vi "test_mergeClusters.vi"(8 "error in (no error)":errorcluster) -> (0 "error out":errorcluster)   [LabVIEW 2020]
uses:
  _built_ppls/OpenVariant.lvlibp
  <vilib>/addons/_JKI Toolkits/Caraya/classes/Test/Test.lvclass
  <vilib>/addons/_JKI Toolkits/Caraya/classes/Assert/Assert.lvclass
  <vilib>/addons/_JKI Toolkits/Caraya/classes/Assert/Assert Equal Value and Type_Variant.vi
panel:
  out "Data out":variant
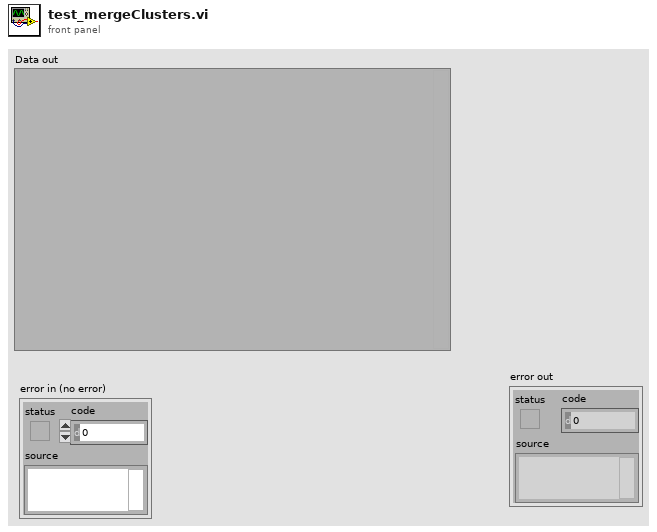
[diagram p1: front panel]
types:
  T1 = cluster{"status":bool, "source":string, "error":errorcluster}
  T2 = cluster{"status":bool, "source":string, "error":cluster{"status":bool, "code":i32, "source":string, "new value":i32}, "code":i32}
  T3 = cluster{"code":i32, "source":string, "error":cluster{"code":i32, "source":string, "new value":i32}}
  T4 = cluster{"status":bool, "code":i32, "source":string, "new value":i32}
  T5 = cluster{"status":bool, "code":i32, "new value":i32}
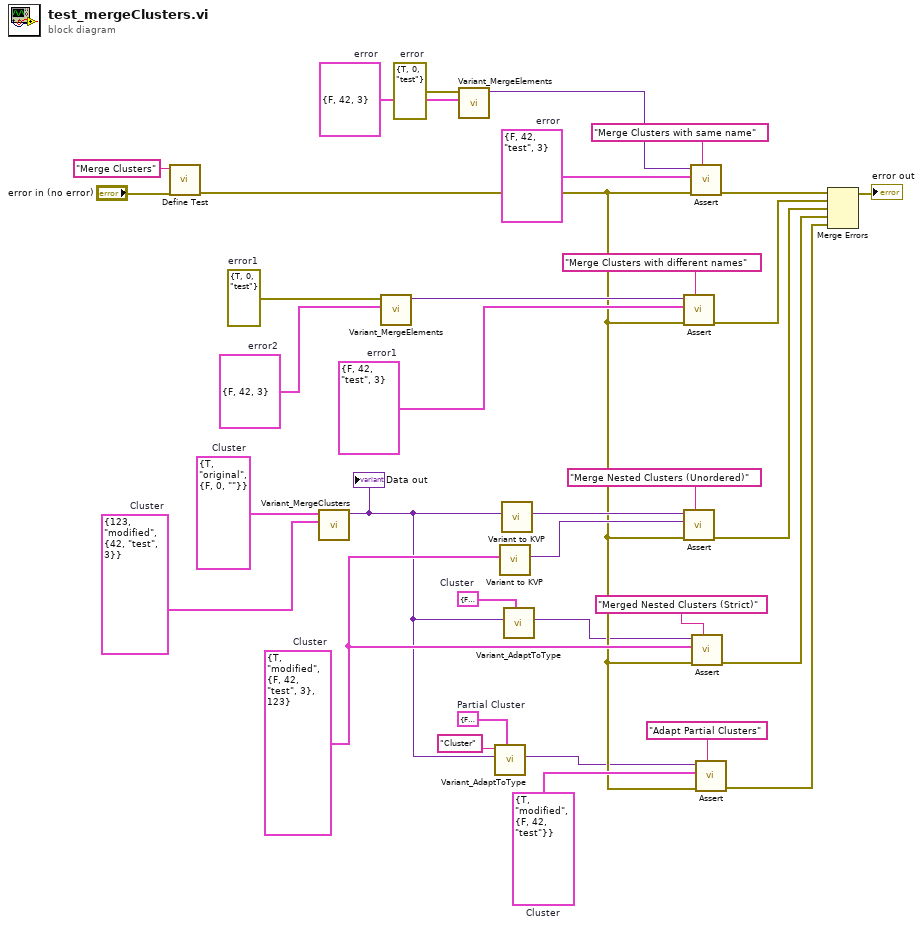
[diagram p0: block diagram]
diagram:
  w4 = T1 {"status"=FALSE, "source"="", "error"={"status"=FALSE, "code"=0, "source"=""}}  # Partial Cluster
  w5 = T2 {"status"=FALSE, "source"="", "error"={"status"=FALSE, "code"=0, "source"="", "new value"=0}, "code"=0}  # Cluster
  w8 = T1 {"status"=TRUE, "source"="modified", "error"={"status"=FALSE, "code"=42, "source"="test"}}  # Cluster
  w12 = T2 {"status"=TRUE, "source"="modified", "error"={"status"=FALSE, "code"=42, "source"="test", "new value"=3}, "code"=123}  # Cluster
  w16 = T3 {"code"=123, "source"="modified", "error"={"code"=42, "source"="test", "new value"=3}}  # Cluster
  w17 = T1 {"status"=TRUE, "source"="original", "error"={"status"=FALSE, "code"=0, "source"=""}}  # Cluster
  w26 = T4 {"status"=FALSE, "code"=42, "source"="test", "new value"=3}  # error1
  w21 = errorcluster {"status"=TRUE, "code"=0, "source"="test"}  # error1
  w20 = T5 {"status"=FALSE, "code"=42, "new value"=3}  # error2
  w31 = T4 {"status"=FALSE, "code"=42, "source"="test", "new value"=3}  # error
  w34 = errorcluster {"status"=TRUE, "code"=0, "source"="test"}  # error
  w28 = T5 {"status"=FALSE, "code"=42, "new value"=3}  # error
  n1 = call <vilib>:"Define Test.vi"("error in (no error)"="error in (no error)", "Label (VI Title)"="Merge Clusters") -> ("error out"=w7:errorcluster)  [unwired: 8 in, 1 out]
  n2 = call "Variant_MergeClusters.vi"("New Element(s)"=w16, "Original Element(s)"=w17) -> ("Merged Cluster"=w3:variant)  [unwired: 9 in]
  "Data out" <- w3
  n3 = call "Variant_MergeElements.vi"("New Element(s)"=w20, "Original Element(s)"=w21) -> ("Merged Elements"=w22:variant)  [unwired: 9 in]
  n4 = call "Variant_MergeElements.vi"("New Element(s)"=w28, "Original Element(s)"=w34) -> ("Merged Elements"=w32:variant)  [unwired: 9 in]
  n5 = call "Variant_AdaptToType.vi"("Default Type"=w4, "Variant"=w3, "Name (Default Type name)"="Cluster" ("Default Value Name (empty: type name)")) -> ("Adapted Variant"=w2:variant)  [unwired: 8 in]
  n6 = call "Variant to KVP.vi"("Variant"=w12) -> ("KVP Dictionary"=w14:variant)  [unwired: 10 in]
  n7 = call "Variant to KVP.vi"("Variant"=w3) -> ("KVP Dictionary"=w15:variant)  [unwired: 10 in]
  n8 = call "Variant_AdaptToType.vi"("Default Type"=w5, "Variant"=w3) -> ("Adapted Variant"=w6:variant)  [unwired: 9 in]
  n9 = call-poly <vilib>:"Assert.vi"("Label"="Merge Clusters with different names" ("Label (VI Title)"), "error in (no error)"=w7, "Y"=w26, "X"=w22) -> ("error out"=w25:errorcluster)  [unwired: 6 in, 1 out]
  n10 = call-poly <vilib>:"Assert.vi"("Label"="Merge Nested Clusters (Unordered)" ("Label (VI Title)"), "error in (no error)"=w7, "Y"=w14, "X"=w15) -> ("error out"=w18:errorcluster)  [unwired: 6 in, 1 out]
  n11 = call-poly <vilib>:"Assert.vi"("Label"="Merge Clusters with same name" ("Label (VI Title)"), "error in (no error)"=w7, "Y"=w31, "X"=w32) -> ("error out"=w24:errorcluster)  [unwired: 6 in, 1 out]
  n12 = call-poly <vilib>:"Assert.vi"("Label"="Merged Nested Clusters (Strict)" ("Label (VI Title)"), "error in (no error)"=w7, "Y"=w12, "X"=w6) -> ("error out"=w11:errorcluster)  [unwired: 6 in, 1 out]
  n13 = call-poly <vilib>:"Assert.vi"("Label"="Adapt Partial Clusters" ("Label (VI Title)"), "error in (no error)"=w7, "Y"=w8, "X"=w2) -> ("error out"=w9:errorcluster)  [unwired: 6 in, 1 out]
  n14 = Merge Errors(w24, w25, w18, w11, w9) -> (→"error out":errorcluster)
